vi "qalibrate_run_function.vi"(10 "Run button ref":refnum<vi>, 11 "function name":string) -> ()   [LabVIEW 2019]
uses:
  qalibrate.vi
  Global.lvlib
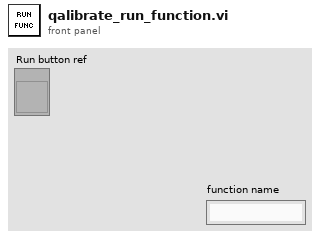
[diagram p1: front panel]
types:
  T1 = enum16{"open", "replace", "create", "open or create", "replace or create", "replace or create with confirmation"}
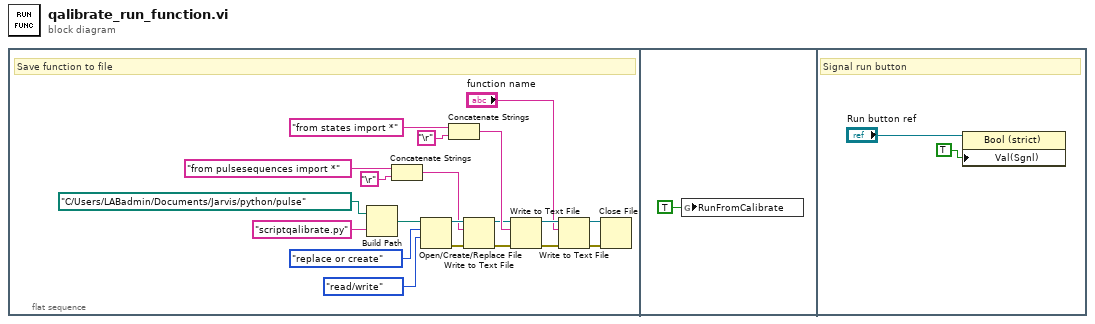
[diagram p0: block diagram]
diagram:
  n1 = flat-sequence {
    frame #0 {
      # "Save function to file"
      n2 = Build Path(base path=path "C:/Users/LABadmin/Documents/Jarvis/python/pulse", name or relative path="scriptqalibrate.py") -> (appended path=w18:path)
      n3 = Concatenate Strings("from pulsesequences import *", "\r") -> (w11:string)
      n4 = Open/Create/Replace File(file path (use dialog)=w18, operation (0:open)=T1."replace or create", access (0:read/write)=enum16{"read/write", "read-only", "write-only"}."read/write") -> (refnum out=w14:refnum<file>, error out=w15:errorcluster)  [unwired: 3 in, 1 out]
      n5 = Concatenate Strings("from states import *", "\r") -> (w8:string)
      n6 = Write to Text File(file (use dialog)=w14, text=w11, error in=w15) -> (refnum out=w7:refnum<file>, error out=w6:errorcluster)  [unwired: 1 in, 1 out]
      n7 = Write to Text File(file (use dialog)=w7, text=w8, error in=w6) -> (refnum out=w5:refnum<file>, error out=w4:errorcluster)  [unwired: 1 in, 1 out]
      n8 = Write to Text File(file (use dialog)=w5, text="function name", error in=w4) -> (refnum out=w3:refnum<file>, error out=w2:errorcluster)  [unwired: 1 in, 1 out]
      n9 = Close File(refnum=w3, error in=w2) -> ()  [unwired: 2 out]
    }
    frame #1 {
      n10 = global write "qalibrate.vi" "RunFromCalibrate"(TRUE ("RunFromCalibrate")) -> ()
    }
    frame #2 {
      # "Signal run button"
      n11 = property class="Bool (strict)"(reference="Run button ref", "Val(Sgnl)"=TRUE ("Value (Signaling)")) -> ()  [unwired: 1 in, 2 out]
    }
  }
